vi "obj_Library Session.vi"(0 "method":T1, 5 "path":path, 7 "argument in (none)":string, 9 "ancillary in (none)":string, 11 "error in (no error)":errorcluster) -> (4 "cleanup/empty?":bool, 8 "argument out":string, 10 "ancillary out":string, 15 "error out":errorcluster)   [LabVIEW 2012]
doc: "Object to assist in the persistence of a session of top-level user interface windows. This object holds the paths of the VIs running in the current session as well as optional arguments per running VI. When the session is stopped, this session data is persisted. When the session is started, the persisted session data is used to re-run all VIs (with optional arguments). An argument is of particular use for discriminating instances of a VI template.\n\nTo support session management, top-level user interface windows must get any arguments passed to them, check if the global session cleanup has been triggered, and delist themselves from the session when they stop running. Any other data that is particular to such a user interface window and is in need of being persisted (its position or the content of certain controls) is the responsibility of that VI itself.\n\nSome master VI is required to start and stop the session. In simple cases, this occurs at application initialization and cleanup respectively. In case of a client able to connect to multiple servers, session starting and stopping should be performed on connecting / disconnecting. Make sure that the persistence path configuration global is set uniquely per connection to prevent session and other persistence data of different servers from getting mixed up."
uses:
  typedefs/t_Library Session Methods.ctl
panel:
  in  "ancillaries persist":string[](array[string])
  in  "arguments persist":string[](array[string])
  in  "paths persist":path[](array[path])
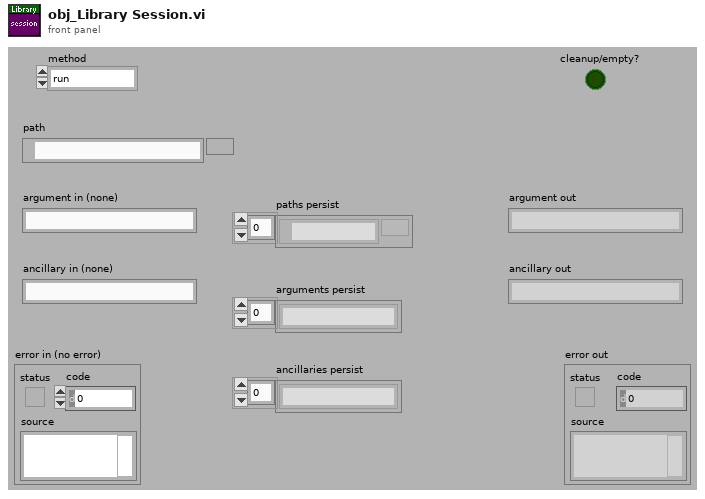
[diagram p1: front panel]
types:
  T1 = typedef "t_Library Session Methods.ctl" = enum16{"run", "get arg", "set arg", "delist", "cleanup?", "start session", "stop session", "list empty?"}
  T2 = enum32{"Bad", "Idle", "Run top level", "Running"}
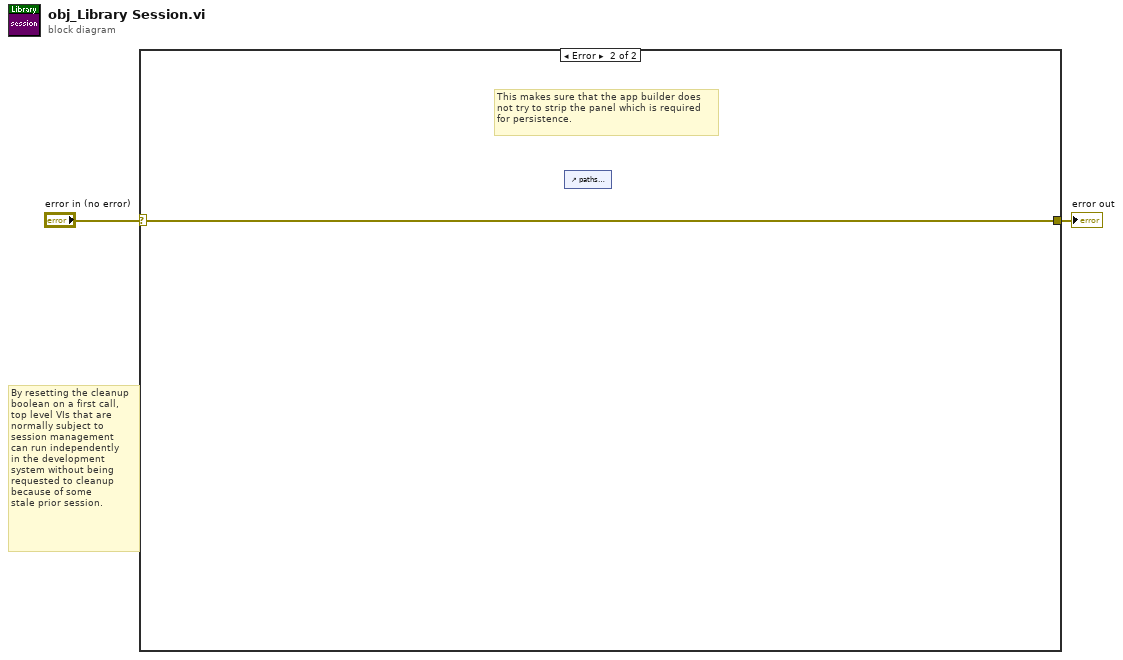
[diagram p0: block diagram]
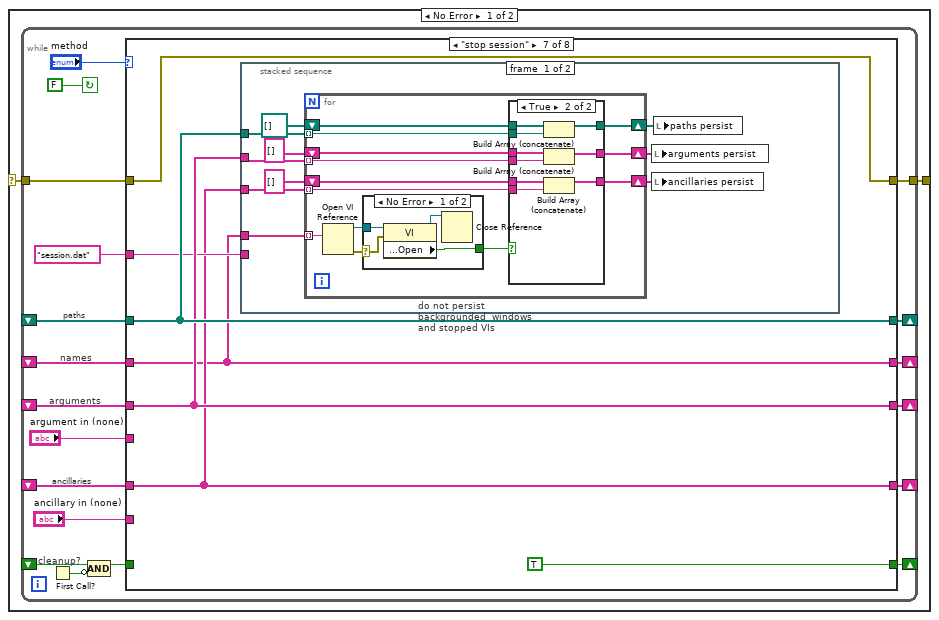
[diagram p2: hidden frame]
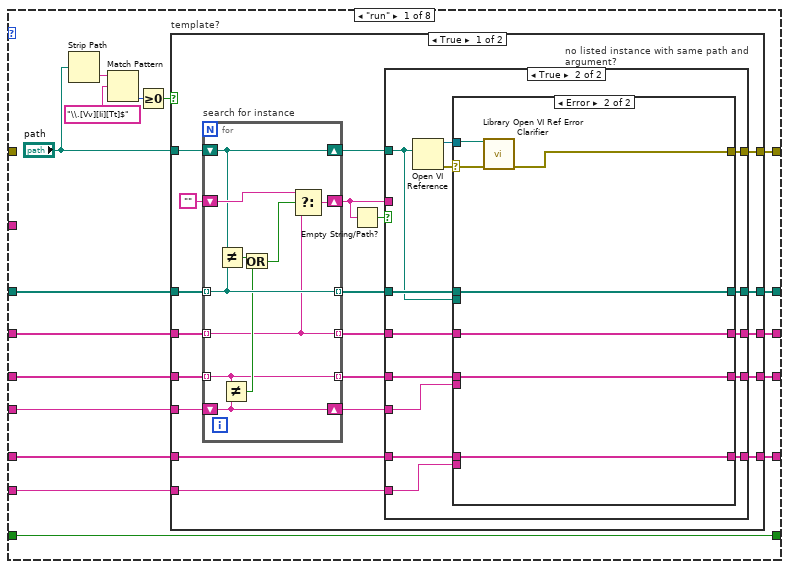
[diagram p3: hidden frame]
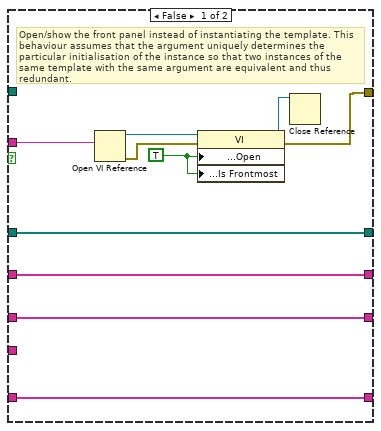
[diagram p4: hidden frame]
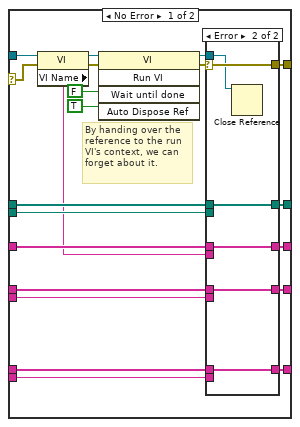
[diagram p5: hidden frame]
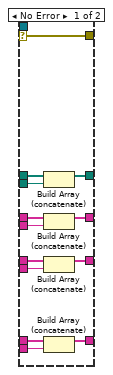
[diagram p6: hidden frame]
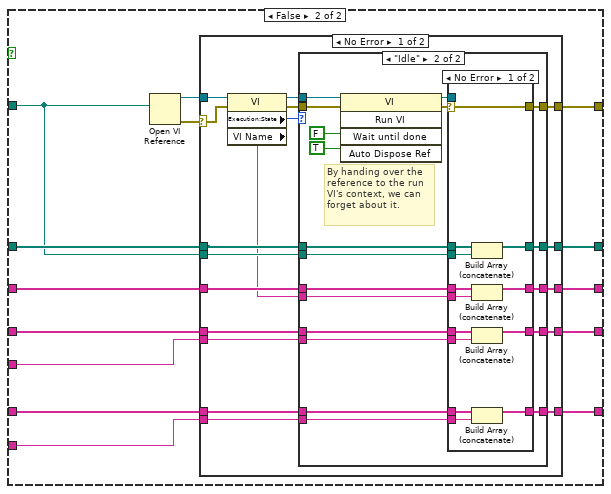
[diagram p7: hidden frame]
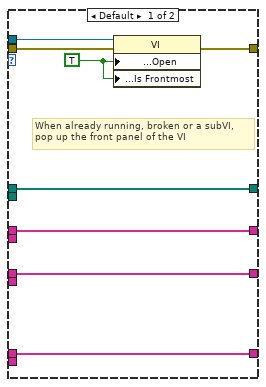
[diagram p8: hidden frame]
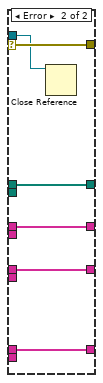
[diagram p9: hidden frame]
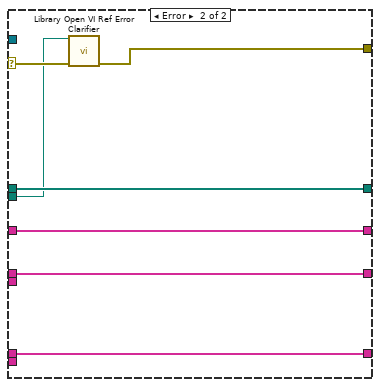
[diagram p10: hidden frame]
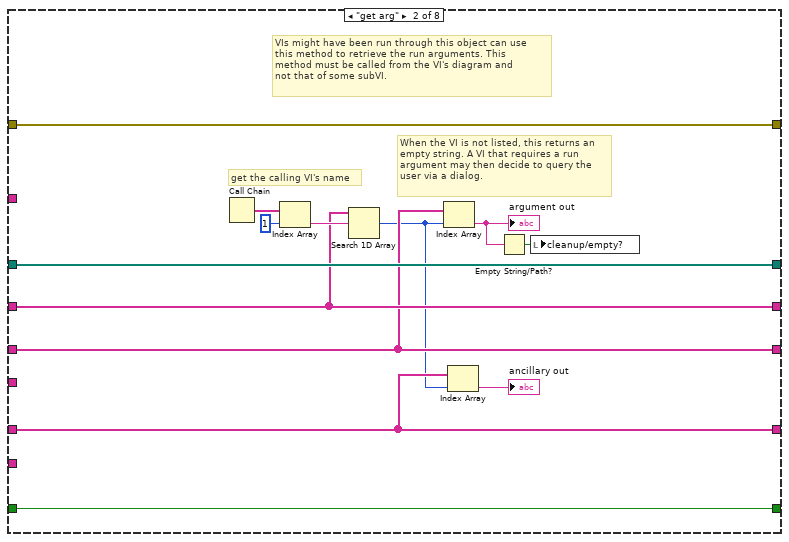
[diagram p11: hidden frame]
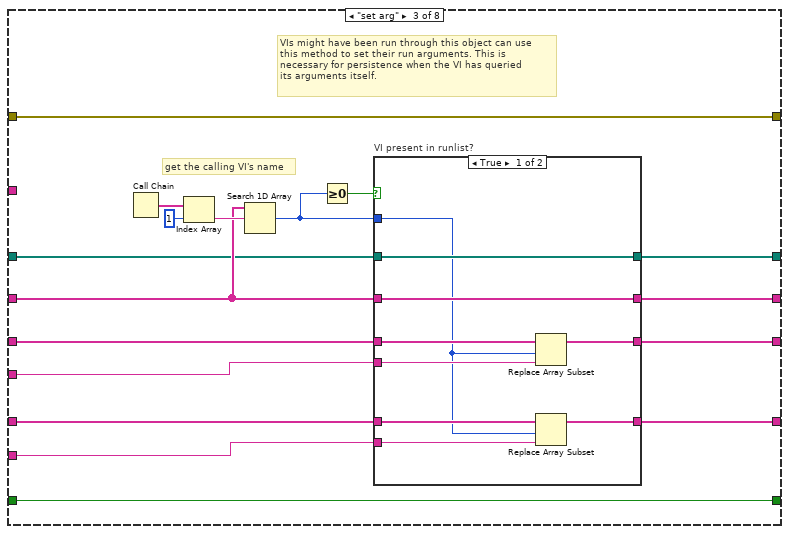
[diagram p12: hidden frame]
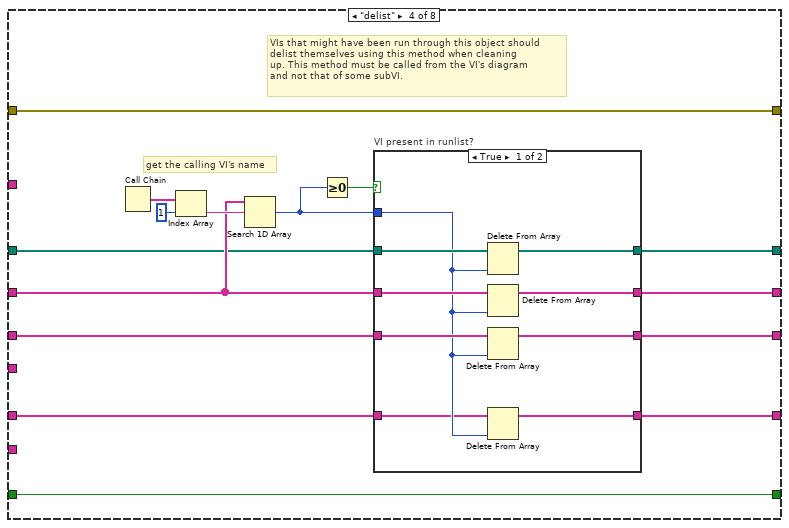
[diagram p14: hidden frame]
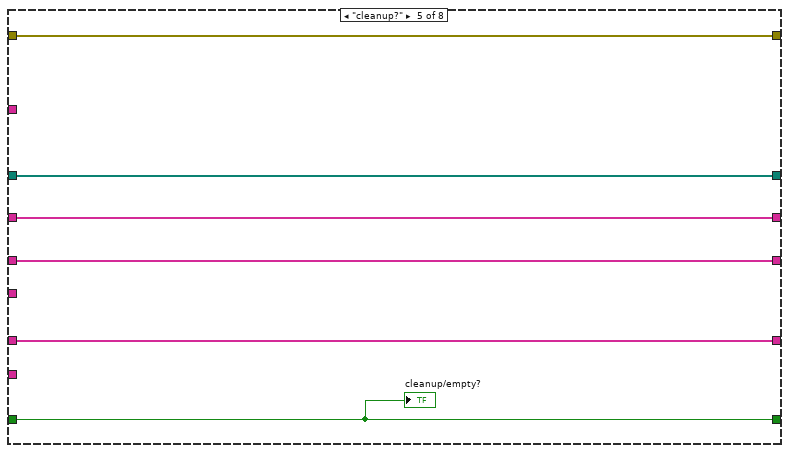
[diagram p16: hidden frame]
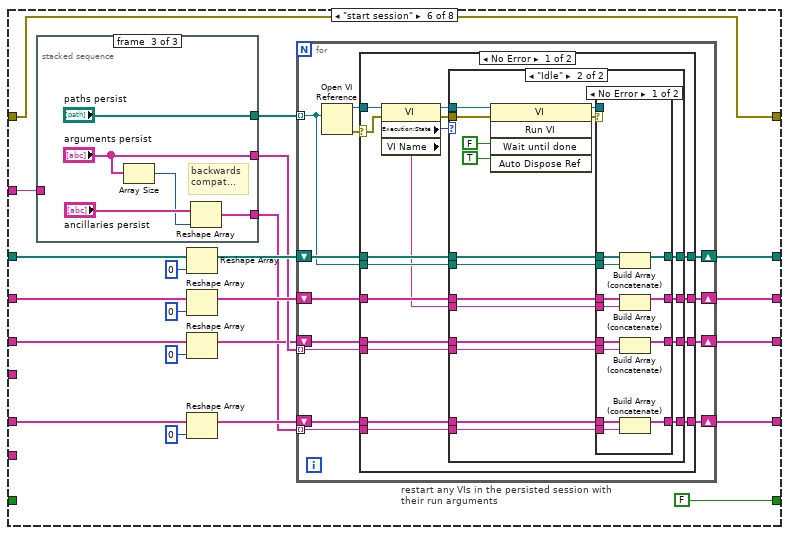
[diagram p17: hidden frame]
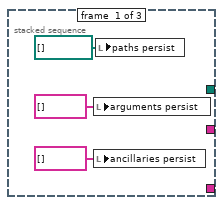
[diagram p18: hidden frame]
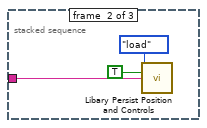
[diagram p19: hidden frame]
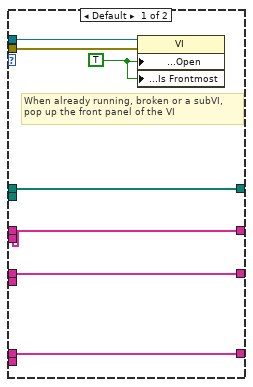
[diagram p20: hidden frame]
diagram:
  # "By resetting the cleanup\nboolean on a first call,\ntop level VIs that are\nnormally subject to\nsession management\ncan run independently\nin the development\nsystem without being\nrequested to cleanup\nbecause of some\nstale prior session."
  n1 = case shown="Error" "error in (no error)" {
    selector: "error in (no error)" -> [w4 w470]
    tunnel: [w3 w470] -> w1
    frame No Error {
      n2 = while {
        shift-right: [w23] -> _
        shift-left: _ -> [w22]
        shift-right: [w20] -> _
        shift-left: _ -> [w21]
        tunnel: w4 -> [w19]
        tunnel: [w18] -> w3
        shift-right: [w17] -> _
        shift-left: _ -> [w10]
        shift-right: [w13] -> _
        shift-left: _ -> [w16]
        shift-right: [w6] -> _
        shift-left: _ -> [w7]
        stop <- FALSE continue-if-true
        # "ancillaries"
        # "cleanup?"
        # "arguments"
        # "names"
        # "paths"
        n3 = First Call?() -> (First Call?: T/F=w8:bool)
        n4 = Compound Arithmetic op=AND(w16, invert w8) -> (w9:bool)
        n5 = case shown="\"stop session\"" "method" {
          tunnel: w22 -> [w38 w234 w250 w277 w302 w324 w418 w465]
          tunnel: [w39 w234 w249 w276 w302 w323 w418 w465] -> w23
          tunnel: [w37 w233 w248 w275 w299 w322 w414 w466] -> w20
          tunnel: w21 -> [w36 w233 w251 w278 w299 w314 w414 w466]
          tunnel: w19 -> [_ w235 w253 w280 w303 w318 w413 w469]
          tunnel: [w40 w235 w253 w280 w303 w318 w413 w469] -> w18
          tunnel: w10 -> [w35 w232 w252 w279 w300 w311 w417 w467]
          tunnel: [w34 w232 w247 w274 w300 w325 w417 w467] -> w17
          tunnel: w9 -> [w33 w236 w243 w281 w301 _ _ w468]
          tunnel: [w33 w236 w243 w281 w301 FALSE TRUE w468] -> w13
          tunnel: "argument in (none)" -> [w32 _ w244 _ _ _ _ _]
          tunnel: "session.dat" ("filename (<window title>.dat)") -> [_ _ _ _ _ w321 w416 _]
          tunnel: w7 -> [w26 w228 w241 w270 w298 w307 w415 w462]
          tunnel: [w25 w228 w242 w271 w298 w306 w415 w462] -> w6
          tunnel: "ancillary in (none)" -> [w24 _ w240 _ _ _ _ _]
          frame "run" {
            n6 = Strip Path(path="path") -> (name=w30:string)  [unwired: 1 out]
            n7 = Match Pattern(string=w30, regular expression="\\.[Vv][Ii][Tt]$") -> (offset past match=w28:i32)  [unwired: 1 in, 3 out]
            n8 = Greater Or Equal To 0?(x=w28) -> (x >= 0?=w27:bool)
            n9 = case "template?" shown="True" w27 {
              tunnel: [w60 w153] -> w40
              tunnel: [w59 w152] -> w39
              tunnel: w38 -> [w56 w151]
              tunnel: [w58 w150] -> w37
              tunnel: w36 -> [w55 w149]
              tunnel: w35 -> [w54 w148]
              tunnel: [w57 w147] -> w34
              tunnel: w32 -> [w49 w146]
              tunnel: "path" -> [w46 w145]
              tunnel: w26 -> [w41 w144]
              tunnel: [w43 w143] -> w25
              tunnel: w24 -> [w42 w142]
              frame True {
                n10 = for "search for instance" {
                  shift-right: [w66] -> w44
                  shift-left: "" -> [w63]
                  tunnel: w56 -> [w70] mode=indexing
                  tunnel: w55 -> [w61] mode=indexing
                  tunnel: w54 -> [w64] mode=indexing
                  tunnel: [w64] -> w53 mode=indexing
                  tunnel: [w61] -> w52 mode=indexing
                  tunnel: [w70] -> w51 mode=indexing
                  shift-right: [w69] -> w48
                  shift-left: w49 -> [w69]
                  shift-right: [w62] -> w45
                  shift-left: w46 -> [w62]
                  n11 = Not Equal?(x=w62, y=w70) -> (x != y?=w68:bool)
                  n12 = Not Equal?(x=w64, y=w69) -> (x != y?=w67:bool)
                  n13 = Or(x=w68, y=w67) -> (x .or. y?=w65:bool)
                  n14 = Select(t=w63, s=w65, f=w61) -> (s? t:f=w66:string)
                }
                n15 = Empty String/Path?(string/path=w44) -> (empty?=w47:bool)
                n16 = case "no listed instance with same path and argument?" shown="True" w47 {
                  tunnel: [w76 w92] -> w60
                  tunnel: [w79 w91] -> w59
                  tunnel: w51 -> [w79 w90]
                  tunnel: [w78 w89] -> w58
                  tunnel: w52 -> [w78 w88]
                  tunnel: w53 -> [w77 w87]
                  tunnel: [w77 w86] -> w57
                  tunnel: w48 -> [_ w85]
                  tunnel: w45 -> [_ w84]
                  tunnel: w44 -> [w80 _]
                  tunnel: w41 -> [w75 w83]
                  tunnel: [w75 w81] -> w43
                  tunnel: w42 -> [_ w82]
                  frame False {
                    w74 = TRUE ("Front Panel Window:Open")
                    # "Open/show the front panel instead of instantiating the template. This behaviour assumes that the argument uniquely determines the particular initialisation of the instance so that two instances of the same template with the same argument are equivalent and thus redundant."
                    n17 = Open VI Reference(vi path=w80) -> (vi reference=w73:refnum<vi>, error out=w72:errorcluster)  [unwired: 5 in]
                    n18 = property class="VI"(reference=w73, error in=w72, "Front Panel Window:Open"=w74, "Front Panel Window:Is Frontmost"=w74) -> (reference out=w71:refnum<vi>, error out=w76:errorcluster)
                    n19 = Close Reference(reference=w71) -> ()  [unwired: 1 in, 1 out]
                  }
                  frame True {
                    n20 = Open VI Reference(vi path=w84) -> (vi reference=w94:refnum<vi>, error out=w93:errorcluster)  [unwired: 5 in]
                    n21 = case shown="Error" w93 {
                      selector: w93 -> [w114 w138]
                      tunnel: w94 -> [w115 _]
                      tunnel: [w111 w137] -> w92
                      tunnel: w90 -> [w105 w141]
                      tunnel: [w110 w141] -> w91
                      tunnel: [w109 w140] -> w89
                      tunnel: w88 -> [w106 w140]
                      tunnel: w87 -> [w107 w139]
                      tunnel: [w108 w139] -> w86
                      tunnel: w84 -> [w104 w136]
                      tunnel: w85 -> [w102 _]
                      tunnel: w83 -> [w97 w135]
                      tunnel: w82 -> [w96 _]
                      tunnel: [w95 w135] -> w81
                      frame No Error {
                        # "By handing over the\nreference to the run\nVI's context, we can\nforget about it."
                        n22 = property class="VI"(reference=w115, error in=w114) -> (reference out=w112:refnum<vi>, error out=w113:errorcluster, "VI Name"=w103:string)
                        n23 = invoke class="VI" method="Run VI"(reference=w112, error in=w113, "Wait until done"=FALSE, "Auto Dispose Ref"=TRUE) -> (reference out=w98:refnum<vi>, error out=w99:errorcluster)  [unwired: 1 in, 3 out]
                        n24 = case shown="Error" w99 {
                          selector: w99 -> [w128 w134]
                          tunnel: [w128 w134] -> w111
                          tunnel: w98 -> [_ w133]
                          tunnel: [w126 w130] -> w110
                          tunnel: [w122 w131] -> w109
                          tunnel: [w120 w132] -> w108
                          tunnel: w107 -> [w121 w132]
                          tunnel: w106 -> [w124 w131]
                          tunnel: w105 -> [w127 w130]
                          tunnel: w104 -> [w125 _]
                          tunnel: w103 -> [w123 _]
                          tunnel: w102 -> [w119 _]
                          tunnel: w97 -> [w118 w129]
                          tunnel: w96 -> [w117 _]
                          tunnel: [w116 w129] -> w95
                          frame No Error {
                            n25 = Build Array (concatenate)(w127, w125) -> (w126:path[])
                            n26 = Build Array (concatenate)(w124, w123) -> (w122:string[])
                            n27 = Build Array (concatenate)(w121, w119) -> (w120:string[])
                            n28 = Build Array (concatenate)(w118, w117) -> (w116:string[])
                          }
                          frame Error {
                            n29 = Close Reference(reference=w133) -> ()  [unwired: 1 in, 1 out]
                          }
                        }
                      }
                      frame Error {
                        n30 = call "Library Open VI Ref Error Clarifier.vi"("VI path"=w136, "called VI error (no error)"=w138) -> ("error out"=w137:errorcluster)  [unwired: 13 in]
                      }
                    }
                  }
                }
              }
              frame False {
                n31 = Open VI Reference(vi path=w145) -> (vi reference=w155:refnum<vi>, error out=w154:errorcluster)  [unwired: 5 in]
                n32 = case shown="No Error" w154 {
                  selector: w154 -> [w172 w223]
                  tunnel: w155 -> [w173 _]
                  tunnel: [w168 w222] -> w153
                  tunnel: w151 -> [w162 w226]
                  tunnel: [w167 w226] -> w152
                  tunnel: [w166 w225] -> w150
                  tunnel: w149 -> [w163 w225]
                  tunnel: w148 -> [w164 w224]
                  tunnel: [w165 w224] -> w147
                  tunnel: w145 -> [w161 w221]
                  tunnel: w146 -> [w159 _]
                  tunnel: w144 -> [w158 w220]
                  tunnel: [w157 w220] -> w143
                  tunnel: w142 -> [w156 _]
                  frame No Error {
                    n33 = property class="VI"(reference=w173, error in=w172) -> (reference out=w169:refnum<vi>, error out=w170:errorcluster, "Execution:State"=w171:T2, "VI Name"=w160:string)
                    n34 = case shown="\"Idle\"" w171 {
                      tunnel: w170 -> [w175 w198]
                      tunnel: w169 -> [w177 w197]
                      tunnel: [w176 w195] -> w168
                      tunnel: [w181 w193] -> w167
                      tunnel: [w180 w192] -> w166
                      tunnel: [w179 w191] -> w165
                      tunnel: w164 -> [w179 w190]
                      tunnel: w163 -> [w180 w189]
                      tunnel: w162 -> [w181 w188]
                      tunnel: w161 -> [_ w187]
                      tunnel: w160 -> [_ w186]
                      tunnel: w159 -> [_ w185]
                      tunnel: w158 -> [w174 w184]
                      tunnel: [w174 w183] -> w157
                      tunnel: w156 -> [_ w182]
                      frame Default {
                        w178 = TRUE ("Front Panel Window:Open")
                        # "When already running, broken or a subVI,\npop up the front panel of the VI"
                        n35 = property class="VI"(reference=w177, error in=w175, "Front Panel Window:Open"=w178, "Front Panel Window:Is Frontmost"=w178) -> (error out=w176:errorcluster)  [unwired: 1 out]
                      }
                      frame "Idle" {
                        # "By handing over the\nreference to the run\nVI's context, we can\nforget about it."
                        n36 = invoke class="VI" method="Run VI"(reference=w197, error in=w198, "Wait until done"=FALSE, "Auto Dispose Ref"=TRUE) -> (reference out=w194:refnum<vi>, error out=w196:errorcluster)  [unwired: 1 in, 3 out]
                        n37 = case shown="No Error" w196 {
                          selector: w196 -> [w213 w219]
                          tunnel: [w213 w219] -> w195
                          tunnel: w194 -> [_ w218]
                          tunnel: [w211 w215] -> w193
                          tunnel: [w207 w216] -> w192
                          tunnel: [w205 w217] -> w191
                          tunnel: w190 -> [w206 w217]
                          tunnel: w189 -> [w209 w216]
                          tunnel: w188 -> [w212 w215]
                          tunnel: w187 -> [w210 _]
                          tunnel: w186 -> [w208 _]
                          tunnel: w185 -> [w204 _]
                          tunnel: w184 -> [w203 w214]
                          tunnel: [w202 w214] -> w183
                          tunnel: w182 -> [w201 _]
                          frame No Error {
                            n38 = Build Array (concatenate)(w212, w210) -> (w211:path[])
                            n39 = Build Array (concatenate)(w209, w208) -> (w207:string[])
                            n40 = Build Array (concatenate)(w206, w204) -> (w205:string[])
                            n41 = Build Array (concatenate)(w203, w201) -> (w202:string[])
                          }
                          frame Error {
                            n42 = Close Reference(reference=w218) -> ()  [unwired: 1 in, 1 out]
                          }
                        }
                      }
                    }
                  }
                  frame Error {
                    n43 = call "Library Open VI Ref Error Clarifier.vi"("VI path"=w221, "called VI error (no error)"=w223) -> ("error out"=w222:errorcluster)  [unwired: 13 in]
                  }
                }
              }
            }
          }
          frame "get arg" {
            # "get the calling VI's name"
            # "When the VI is not listed, this returns an\nempty string. A VI that requires a run\nargument may then decide to query the\nuser via a dialog."
            # "VIs might have been run through this object can use\nthis method to retrieve the run arguments. This\nmethod must be called from the VI's diagram and\nnot that of some subVI."
            n44 = Call Chain() -> (call chain=w238:string[])
            n45 = Index Array(array=w238, index=1) -> (element=w237:string)
            n46 = Search 1D Array(1D array=w233, element=w237) -> (index of element=w227:i32)  [unwired: 1 in]
            n47 = Index Array(array=w232, index=w227) -> (element=w231:string)
            "argument out" <- w231
            n48 = Index Array(array=w228, index=w227) -> (element=→"ancillary out":string)
            n49 = Empty String/Path?(string/path=w231) -> (empty?=w230:bool)
            n50 = local write "cleanup/empty?"(w230) -> ()
          }
          frame "set arg" {
            # "get the calling VI's name"
            # "VIs might have been run through this object can use\nthis method to set their run arguments. This is\nnecessary for persistence when the VI has queried\nits arguments itself."
            n51 = Call Chain() -> (call chain=w255:string[])
            n52 = Index Array(array=w255, index=1) -> (element=w254:string)
            n53 = Search 1D Array(1D array=w251, element=w254) -> (index of element=w245:i32)  [unwired: 1 in]
            n54 = Greater Or Equal To 0?(x=w245) -> (x >= 0?=w246:bool)
            n55 = case "VI present in runlist?" shown="True" w246 {
              tunnel: w250 -> [w263 w269]
              tunnel: w251 -> [w262 w268]
              tunnel: w252 -> [w265 w267]
              tunnel: [w263 w269] -> w249
              tunnel: [w262 w268] -> w248
              tunnel: [w264 w267] -> w247
              tunnel: w245 -> [w257 _]
              tunnel: w244 -> [w261 _]
              tunnel: [w260 w266] -> w242
              tunnel: w241 -> [w259 w266]
              tunnel: w240 -> [w258 _]
              frame True {
                n56 = Replace Array Subset(array=w265, new element=w261, index=w257) -> (w264:string[])
                n57 = Replace Array Subset(array=w259, new element=w258, index=w257) -> (w260:string[])
              }
              frame False {
              }
            }
          }
          frame "delist" {
            # "get the calling VI's name"
            # "VIs that might have been run through this object should\ndelist themselves using this method when cleaning\nup. This method must be called from the VI's diagram\nand not that of some subVI."
            n58 = Call Chain() -> (call chain=w283:string[])
            n59 = Index Array(array=w283, index=1) -> (element=w282:string)
            n60 = Search 1D Array(1D array=w278, element=w282) -> (index of element=w272:i32)  [unwired: 1 in]
            n61 = Greater Or Equal To 0?(x=w272) -> (x >= 0?=w273:bool)
            n62 = case "VI present in runlist?" shown="True" w273 {
              tunnel: w277 -> [w293 w297]
              tunnel: w278 -> [w291 w296]
              tunnel: w279 -> [w289 w295]
              tunnel: [w292 w297] -> w276
              tunnel: [w290 w296] -> w275
              tunnel: [w288 w295] -> w274
              tunnel: w272 -> [w286 _]
              tunnel: [w287 w294] -> w271
              tunnel: w270 -> [w285 w294]
              frame True {
                n63 = Delete From Array(array=w293, index=w286) -> (array with subset deleted=w292:path[])  [unwired: 1 in, 1 out]
                n64 = Delete From Array(array=w291, index=w286) -> (array with subset deleted=w290:string[])  [unwired: 1 in, 1 out]
                n65 = Delete From Array(array=w289, index=w286) -> (array with subset deleted=w288:string[])  [unwired: 1 in, 1 out]
                n66 = Delete From Array(array=w285, index=w286) -> (array with subset deleted=w287:string[])  [unwired: 1 in, 1 out]
              }
              frame False {
              }
            }
          }
          frame "cleanup?" {
            "cleanup/empty?" <- w301
          }
          frame "start session" {
            n67 = stacked-sequence {
              tunnel: w321 -> [_ w330 _]
              tunnel: [_ _ "paths persist"] -> w320
              tunnel: [_ _ "arguments persist"] -> w310
              tunnel: [_ _ w332] -> w304
              frame #0 {
                n68 = local write "arguments persist"(string[] [] ("arguments persist")) -> ()
                n69 = local write "ancillaries persist"(string[] [] ("arguments persist")) -> ()
                n70 = local write "paths persist"(path[] [] ("paths persist")) -> ()
              }
              frame #1 {
                n71 = call "Libary Persist Position and Controls.vi"("action"=enum16{"save", "load"}."load", "do not persist bounds (false)"=TRUE ("do not persist position (false)"), "filename (<window title hash>.dat)"=w330) -> ()  [unwired: 11 in, 2 out]
              }
              frame #2 {
                # "backwards\ncompat..."
                n72 = Array Size(array="arguments persist") -> (size(s)=w333:i32)
                n73 = Reshape Array("ancillaries persist", w333) -> (w332:string[])
              }
            }
            n74 = Reshape Array(w324, 0 ("dimension size")) -> (w317:path[])
            n75 = Reshape Array(w314, 0 ("dimension size")) -> (w313:string[])
            n76 = Reshape Array(w311, 0 ("dimension size")) -> (w309:string[])
            n77 = Reshape Array(w307, 0 ("dimension size")) -> (w305:string[])
            n78 = for "restart any VIs in the persisted session with their run arguments" {
              shift-right: [w345] -> w325
              shift-left: w309 -> [w340]
              shift-right: [w346] -> w322
              shift-left: w313 -> [w343]
              shift-right: [w347] -> w323
              shift-left: w317 -> [w344]
              tunnel: w320 -> [w342] mode=indexing
              tunnel: w310 -> [w341] mode=indexing
              shift-right: [w338] -> w306
              shift-left: w305 -> [w339]
              tunnel: w304 -> [w337] mode=indexing
              n79 = Open VI Reference(vi path=w342) -> (vi reference=w349:refnum<vi>, error out=w348:errorcluster)  [unwired: 5 in]
              n80 = case shown="No Error" w348 {
                selector: w348 -> [w365 _]
                tunnel: w349 -> [w366 _]
                tunnel: w344 -> [w356 w412]
                tunnel: [w361 w412] -> w347
                tunnel: [w360 w411] -> w346
                tunnel: w343 -> [w357 w411]
                tunnel: w340 -> [w358 w410]
                tunnel: [w359 w410] -> w345
                tunnel: w342 -> [w355 _]
                tunnel: w341 -> [w353 _]
                tunnel: w339 -> [w352 w409]
                tunnel: [w351 w409] -> w338
                tunnel: w337 -> [w350 _]
                frame No Error {
                  n81 = property class="VI"(reference=w366, error in=w365) -> (reference out=w362:refnum<vi>, error out=w363:errorcluster, "Execution:State"=w364:T2, "VI Name"=w354:string)
                  n82 = case shown="\"Idle\"" w364 {
                    tunnel: w363 -> [w368 w389]
                    tunnel: w362 -> [w369 w388]
                    tunnel: [w373 w385] -> w361
                    tunnel: [w372 w384] -> w360
                    tunnel: [w371 w383] -> w359
                    tunnel: w358 -> [w371 w382]
                    tunnel: w357 -> [w372 w381]
                    tunnel: w356 -> [w373 w380]
                    tunnel: w355 -> [_ w379]
                    tunnel: w354 -> [_ w378]
                    tunnel: w353 -> [_ w377]
                    tunnel: w352 -> [w367 w376]
                    tunnel: [w367 w375] -> w351
                    tunnel: w350 -> [_ w374]
                    frame Default {
                      w370 = TRUE ("Front Panel Window:Open")
                      # "When already running, broken or a subVI,\npop up the front panel of the VI"
                      n83 = property class="VI"(reference=w369, error in=w368, "Front Panel Window:Open"=w370, "Front Panel Window:Is Frontmost"=w370) -> ()  [unwired: 2 out]
                    }
                    frame "Idle" {
                      n84 = invoke class="VI" method="Run VI"(reference=w388, error in=w389, "Wait until done"=FALSE, "Auto Dispose Ref"=TRUE) -> (reference out=w386:refnum<vi>, error out=w387:errorcluster)  [unwired: 1 in, 3 out]
                      n85 = case shown="No Error" w387 {
                        tunnel: w386 -> [_ w408]
                        tunnel: [w402 w405] -> w385
                        tunnel: [w398 w406] -> w384
                        tunnel: [w396 w407] -> w383
                        tunnel: w382 -> [w397 w407]
                        tunnel: w381 -> [w400 w406]
                        tunnel: w380 -> [w403 w405]
                        tunnel: w379 -> [w401 _]
                        tunnel: w378 -> [w399 _]
                        tunnel: w377 -> [w395 _]
                        tunnel: w376 -> [w394 w404]
                        tunnel: [w393 w404] -> w375
                        tunnel: w374 -> [w392 _]
                        frame No Error {
                          n86 = Build Array (concatenate)(w403, w401) -> (w402:path[])
                          n87 = Build Array (concatenate)(w400, w399) -> (w398:string[])
                          n88 = Build Array (concatenate)(w397, w395) -> (w396:string[])
                          n89 = Build Array (concatenate)(w394, w392) -> (w393:string[])
                        }
                        frame Error {
                          n90 = Close Reference(reference=w408) -> ()  [unwired: 1 in, 1 out]
                        }
                      }
                    }
                  }
                }
                frame Error {
                }
              }
            }
          }
          frame "stop session" {
            n91 = stacked-sequence {
              tunnel: w418 -> [w428 _]
              tunnel: w417 -> [w425 _]
              tunnel: w416 -> [_ w459]
              tunnel: w415 -> [w423 _]
              tunnel: w414 -> [w429 _]
              frame #0 {
                n92 = for "do not persist backgrounded  windows and stopped VIs" {
                  tunnel: w429 -> [w440] mode=indexing
                  shift-right: [w436] -> w426
                  shift-left: path[] [] -> [w437]
                  tunnel: w428 -> [w438] mode=indexing
                  shift-right: [w433] -> w422
                  shift-left: string[] [] -> [w434]
                  tunnel: w425 -> [w435] mode=indexing
                  tunnel: w423 -> [w432] mode=indexing
                  shift-right: [w430] -> w421
                  shift-left: string[] [] -> [w431]
                  n93 = Open VI Reference(vi path=w440) -> (vi reference=w441:refnum<vi>, error out=w442:errorcluster)  [unwired: 5 in]
                  n94 = case shown="No Error" w442 {
                    selector: w442 -> [w456 _]
                    tunnel: w441 -> [w458 _]
                    tunnel: [w455 _] -> w439
                    frame No Error {
                      n95 = property class="VI"(reference=w458, error in=w456) -> (reference out=w457:refnum<vi>, "Front Panel Window:Open"=w455:bool)  [unwired: 1 out]
                      n96 = Close Reference(reference=w457) -> ()  [unwired: 1 in, 1 out]
                    }
                    frame Error {
                    }
                  }
                  n97 = case shown="True" w439 {
                    tunnel: w438 -> [_ w454]
                    tunnel: w437 -> [w445 w453]
                    tunnel: [w445 w452] -> w436
                    tunnel: w435 -> [_ w451]
                    tunnel: w434 -> [w443 w450]
                    tunnel: [w443 w449] -> w433
                    tunnel: w432 -> [_ w448]
                    tunnel: w431 -> [w444 w447]
                    tunnel: [w444 w446] -> w430
                    frame False {
                    }
                    frame True {
                      n98 = Build Array (concatenate)(w453, w454) -> (w452:path[])
                      n99 = Build Array (concatenate)(w450, w451) -> (w449:string[])
                      n100 = Build Array (concatenate)(w447, w448) -> (w446:string[])
                    }
                  }
                }
                n101 = local write "arguments persist"(w422) -> ()
                n102 = local write "ancillaries persist"(w421) -> ()
                n103 = local write "paths persist"(w426) -> ()
              }
              frame #1 {
                n104 = call "Libary Persist Position and Controls.vi"("action"=enum16{"save", "load"}."save", "do not persist bounds (false)"=TRUE ("do not persist position (false)"), "filename (<window title hash>.dat)"=w459) -> ()  [unwired: 11 in, 2 out]
              }
            }
          }
          frame "list empty?" {
            # "This allows the client VI to\nwait around until all VIs in\nthe session have delisted\nthemselves."
            n105 = Array Size(array=w465) -> (size(s)=w463:i32)
            n106 = Equal To 0?(x=w463) -> (x = 0?=w464:bool)
            n107 = local write "cleanup/empty?"(w464) -> ()
          }
        }
      }
    }
    frame Error {
      # "This makes sure that the app builder does\nnot try to strip the panel which is required\nfor persistence."
      n108 = control-ref of="paths persist"() -> ()  [unwired: 1 out]
    }
  }
  "error out" <- w1
